vi "Configure FreeRunning TimerDRV.vi"(8 "error in (no error)":errorcluster, 10 "Target Type":T1, 11 "TimerDRV in":refnum<class "TimerDRV.lvclass">) -> (0 "error out":errorcluster, 3 "TimerDRV out":refnum<class "TimerDRV.lvclass">)   [LabVIEW 2019, in "TimingDRV Engine.lvlib" / "TimerDRV.lvclass"]
uses:
  TimerDRV.lvclass
  TypeDefs/Target Type.ctl
  TimerDRV.lvclass/TimerDRV.ctl
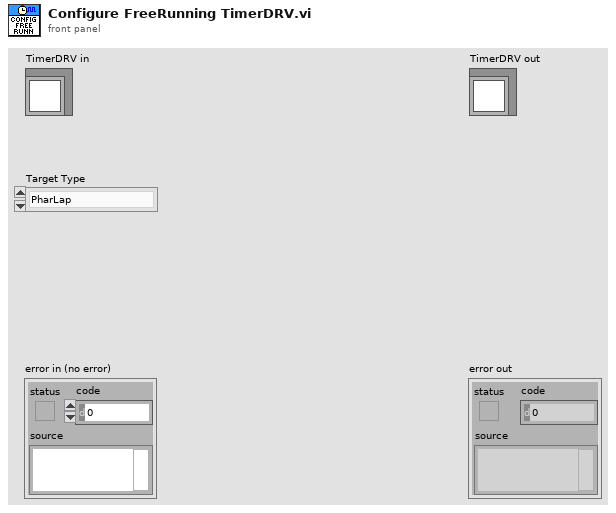
[diagram p1: front panel]
types:
  T1 = typedef "TimingDRV Engine.lvlib/TimerDRV.lvclass/Target Type.ctl" = enum16{"PharLap", "VxWorks", "Windows", "Linux_32_ARM", "Linux_x64"}
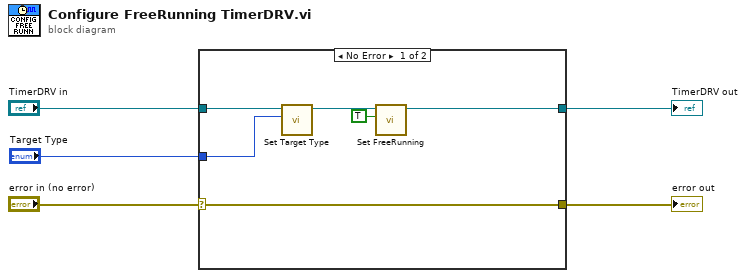
[diagram p0: block diagram]
diagram:
  n1 = case shown="No Error" "error in (no error)" {
    selector: "error in (no error)" -> [w11 w13]
    tunnel: [w11 w13] -> w4
    tunnel: [w10 w12] -> w2
    tunnel: "TimerDRV in" -> [w8 w12]
    tunnel: "Target Type" -> [w6 _]
    frame No Error {
      n2 = call "Set Target Type.vi"("Target Type"=w6, "TimerDRV in"=w8) -> ("TimerDRV out"=w7:refnum<class "TimerDRV.lvclass">)  [unwired: 9 in]
      n3 = call "Set FreeRunning.vi"("FreeRunning"=TRUE, "TimerDRV in"=w7) -> ("TimerDRV out"=w10:refnum<class "TimerDRV.lvclass">)  [unwired: 9 in]
    }
    frame Error {
    }
  }
  "error out" <- w4
  "TimerDRV out" <- w2
